vi "GUI_HTU_Laser_Control_Center.vi"() -> ()   [LabVIEW 2020]
uses:
  Shared/GUI_Template/GUI_master/tcp_new_data_event.ctl
  Shared/GUI_Template/GUI_master/tcp new data cluster.ctl
  GUI_TestStand/Fire button.ctl
panel:
  in  "Open Gaia South Shutter":bool caption="Open gaia North"
  in  "Open Gaia North Shutter":bool caption="Open gaia North"
  in  "Gaia shutter enable":bool caption="Enable gaia \nshutters"
  out "Laser on target":bool
  in  "GUIdevice 28":string="U_MI_FineFilters"
  in  "pos.Channel0::28":enum16{"1", "2", "3", "4", "5", "6"}(ring) caption="Fine Filters"
  in  "DO.Ch9::22":enum16{"off", "on"}(ring) caption="Aline2"
  in  "SoftwareVars.Ch1::22":enum16{"off", "on"}(ring) caption="Autopurge"
  in  "DO.Ch8::22":enum16{"off", "on"}(ring) caption="Aline 3"
  in  "DO.Ch7::22":enum16{"off", "on"}(ring) caption="DC Phos"
  in  "auto purge":bool=TRUE
  in  "purge":bool caption="Purge"
  in  "DO.Ch6::22":enum16{"off", "on"}(ring) caption="purge"
  out "AI_mean.Channel 1::27":dbl caption="Energy (nJ)" min=0.0 max=0.0 format="%.3f"
  out "AI_mean.Channel 0::27":dbl caption="Energy (nJ)" min=0.0 max=0.0 format="%.3f"
  in  "GUIdevice 27":string="U_VacuumGauge"
  out "ACavePressure":dbl format="%#_3g"
  out "BCavePressure":dbl format="%#_3g"
  in  "DigitalOutput.Channel 7::18":enum16{"off", "on"}(ring) caption="Visa9"
  in  "DigitalOutput.Channel 7::25":enum16{"off", "on"}(ring) caption="Visa1"
  in  "DigitalOutput.Channel 6::25":enum16{"off", "on"}(ring) caption="Visa2"
  in  "DigitalOutput.Channel 5::25":enum16{"off", "on"}(ring) caption="Visa3"
  in  "DigitalOutput.Channel 4::25":enum16{"off", "on"}(ring) caption="Visa4"
  in  "DigitalOutput.Channel 3::25":enum16{"off", "on"}(ring) caption="Visa5"
  in  "DigitalOutput.Channel 2::25":enum16{"off", "on"}(ring) caption="Visa6"
  in  "DigitalOutput.Channel 1::25":enum16{"off", "on"}(ring) caption="Visa7"
  in  "DigitalOutput.Channel 0::25":enum16{"off", "on"}(ring) caption="Visa8"
  in  "DigitalOutput.Channel 7::23":enum16{"off", "on"}(ring) caption="Aline1"
  in  "DO.Ch5::22":enum16{"off", "on"}(ring) caption="Beam \nDump"
  in  "DO.Ch4::22":enum16{"off", "on"}(ring) caption="Phos1"
  in  "DO.Ch3::22":enum16{"off", "on"}(ring) caption="MI Wedge"
  in  "DO.Ch2::22":enum16{"off", "on"}(ring) caption="Slit"
  in  "DO.Ch1::22":enum16{"off", "on"}(ring) caption="OAPin2"
  in  "GUIdevice 22":string="U_PLC"
  in  "Position.Channel 8::2":T1(ring) caption="TC phos"
  in  "pos.Channel1::5":enum16{"1", "2", "3", "4", "5", "6"}(ring) caption="HASO"
  in  "pos.Channel0::19":enum16{"1", "2", "3", "4", "5", "6"}(ring) caption="Grating \nCam"
  in  "GUIdevice 19":string="U_FilterWheel_02"
  in  "Delay.Ch B::10":dbl caption="OPening time" min=0.0 max=0.1 format="%#_6p"
  in  "Amplitude.Ch AB::10":dbl caption="Amplitude Jet trigger" min=0.5 max=5.0 format="%.1f"
  in  "DO.Ch10::22":enum16{"off", "on"}(ring) caption="CTR"
  in  "GUIdevice 17":string="U_Hexapod"
  in  "Position.Channel 9::1":T1(ring) caption="Amp 4 dump"
  in  "Position.Channel 10::1":T1(ring) caption="Revo-South Shutter"
  in  "Position.Channel 7::1":T1(ring) caption="Gaia Beamblock 2-North"
  in  "Position.Channel 8::1":T1(ring) caption="Gaia Beamblock 2-South"
  out "Delay.Ch B::10":dbl caption="Opening \ntime (s)" min=0.0 max=0.1 format="%#_6p"
  in  "Set opening time (s)":dbl
  in  "Jet enable":bool caption="Jet Enable"
  in  "pos.Channel3::5":enum16{"1", "2", "3", "4", "5", "6"}(ring) caption="Probe"
  in  "pos.Channel2::5":enum16{"1", "2", "3", "4", "5", "6"}(ring) caption="Ghost\npulsed"
  in  "AnalogOutput.Channel 1::8":dbl caption="Pressure Control Voltage (V)" min=0.0 max=10.0
  in  "Position.Axis 3::7":dbl caption="Jet_Z" min=0.0 max=25.0
  in  "Position.Axis 2::7":dbl caption="Jet_Y" min=-25.0 max=0.0
  in  "Position.Axis 1::7":dbl caption="Jet_X" min=0.0 max=25.0
  in  "pos.Channel0::5":enum16{"1", "2", "3", "4", "5", "6"}(ring) caption="Coarse Filters"
  in  "Position.Channel 6::1":T1(ring) caption="Gaia Beamblock 3-North"
  in  "Position.Channel 5::1":T1(ring) caption="Gaia Beamblock 4-North"
  in  "Position.Channel 4::1":T1(ring) caption="Gaia Stop South"
  in  "Position.Channel 3::1":T1(ring) caption="Gaia Stop North"
  in  "Position.Channel 2::1":T1(ring) caption="Gaia Beamblock 3-South"
  in  "Position.Channel 1::1":T1(ring) caption="Gaia Beamblock 4-South"
  in  "GUIdevice 8":string="U_HP_Daq"
  in  "GUIdevice 5":string="U_FilterWheel_01"
  in  "Fire Button":T2=TRUE
  out "error IO 2":errorcluster
  out "Amplitude.Ch AB::10":dbl caption="Amplitude\n Jet trigger" min=0.5 max=5.0 format="%.1f"
  out "fire::10":string
  out "tcp data event":T3
  in  "UDP error message":string
  in  "GUIdevice 7":string="U_ESP_JetXYZ"
  in  "GUIdevice 2":string="U_1Wire_Bcave"
  in  "GUIdevice 10":string="U_DG645_ShotControl"
  in  "GUIdevice 1":string="U_1Wire_148"
  in  "Step size":dbl min=-22.0 max=22.0 format="%.5f"
  in  "wangle::17":dbl caption="w" min=-7.5 max=7.5 step=0.01 format="%.5f"
  in  "vangle::17":dbl caption="v" min=-7.5 max=7.5 step=0.01 format="%.5f"
  in  "uangle::17":dbl caption="u" min=-7.5 max=7.5 step=0.01 format="%.5f"
  in  "ypos::17":dbl caption="y" min=-24.0 max=24.0 step=0.01 format="%.5f"
  in  "zpos::17":dbl caption="z" min=-10.0 max=10.0 step=0.01 format="%.5f"
  in  "xpos::17":dbl caption="x" min=-20.0 max=20.0 step=0.01 format="%.5f"
  in  "Jet trigger":bool caption="Jet Trigger"
  in  "Delay.Ch C::10":dbl caption="Jet timing (s)" min=-0.1 max=0.1 format="%#_6p"
  in  "stop":bool
  # "HTU CONTROL CENTER"
  # "GAIA Flippers"
  # "B-Cave Laser Status"
  # "Jet Stages"
  # "Energy"
  # "Mode Imager"
  # "Jet timing"
  # "Hexapod"
  # "\"+x\" is laser propagation direction\n\"+y\" is toward parking lot\n\"+z\" is up"
  # "Extra Flippers"
  # "Valve Control"
  # "Filters"
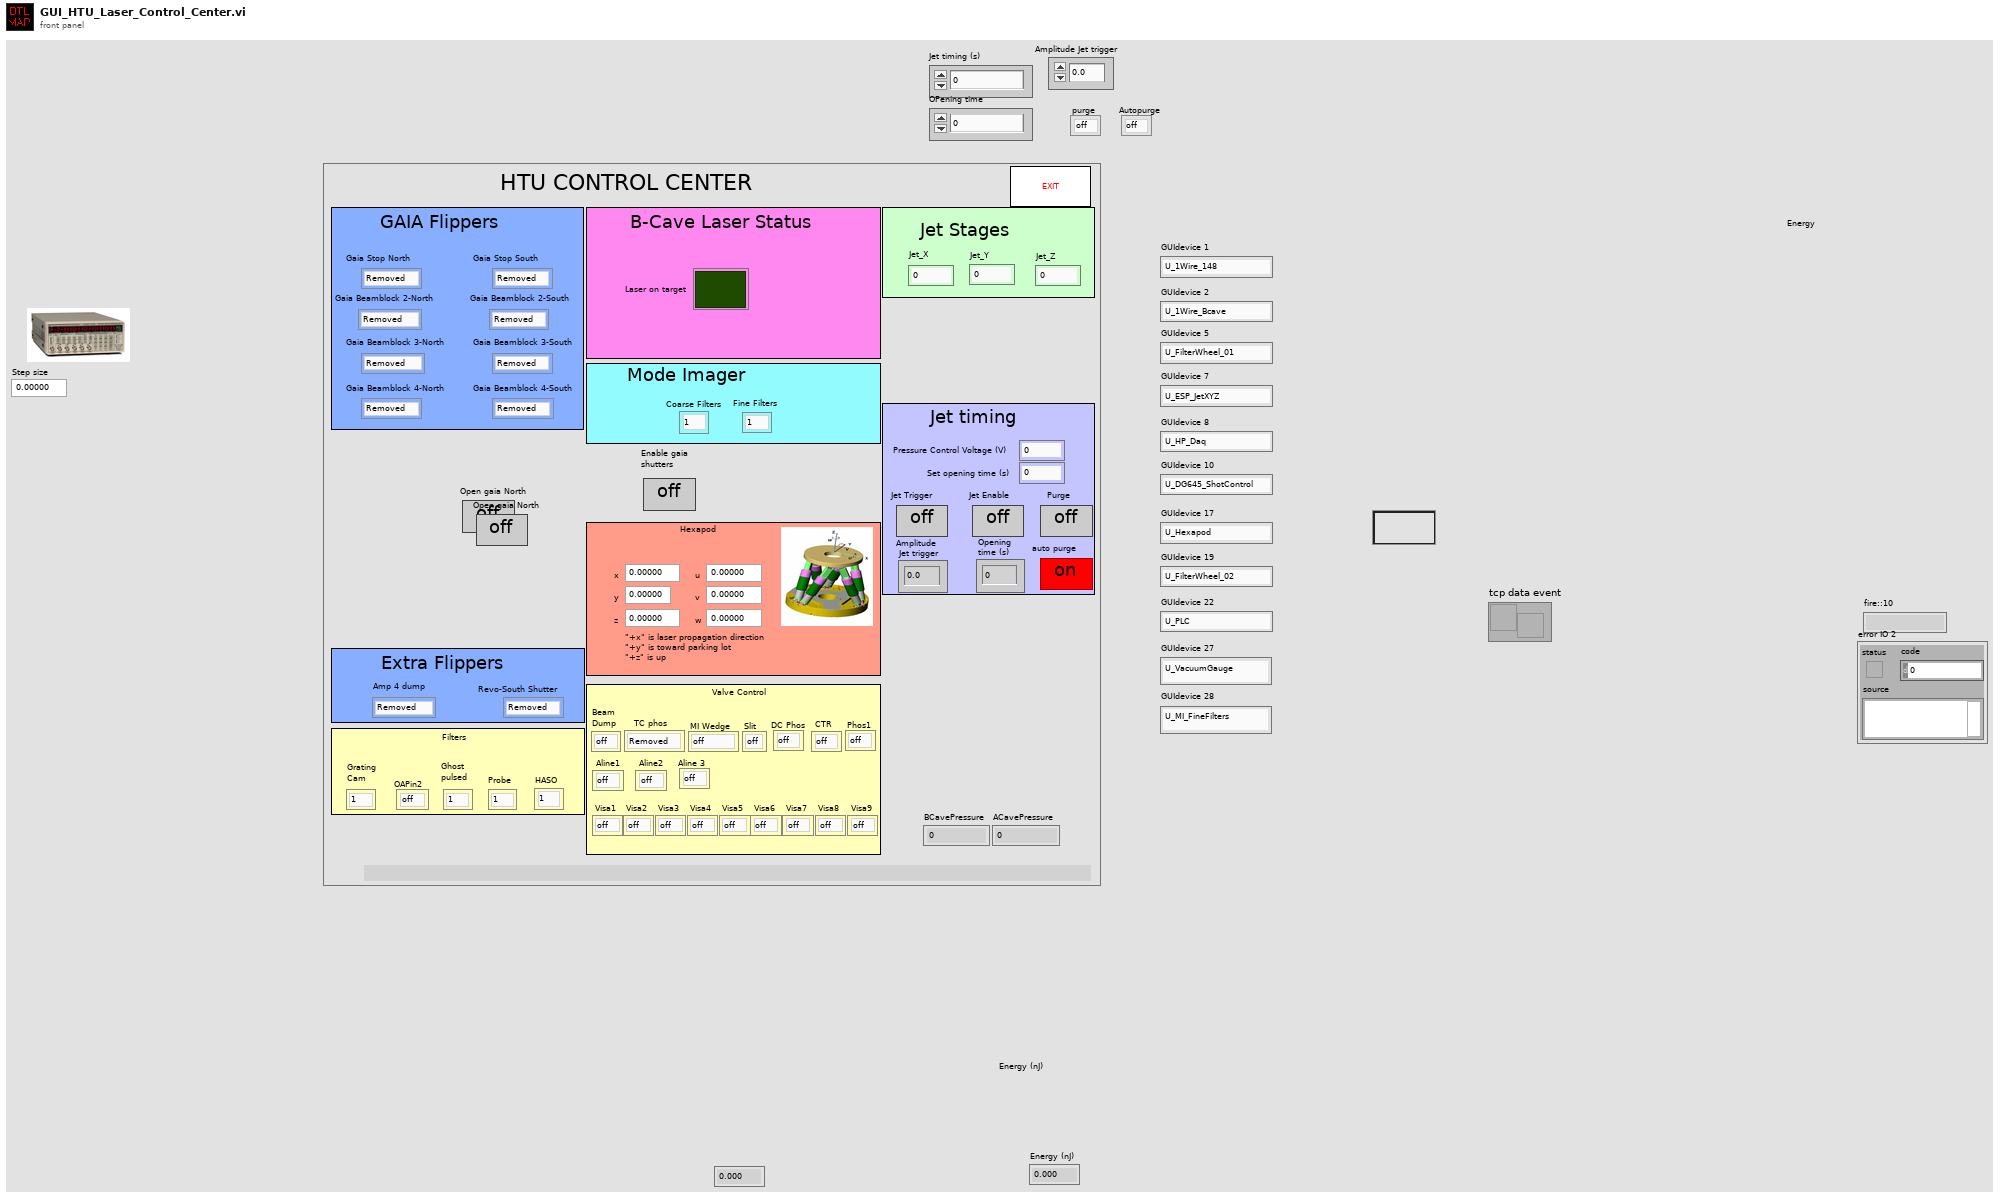
[diagram p1: front panel]
types:
  T1 = enum16{"Removed", "Inserted", "Unknown", "Moving"}
  T2 = typedef "Fire button.ctl" = bool
  T3 = typedef "tcp_new_data_event.ctl" = refnum<user-event>
  T4 = typedef "tcp new data cluster.ctl" = cluster{"EventEnum":enum16{"new data", "connection status update"}, "Device name":string}
  T5 = enum32{"invalid app kind", "Development System", "Run Time System", "Student Edition", "Embedded LabVIEW", "Evaluation", "Custom"}
  T6 = enum32{"Invalid", "Standard", "Closed", "Hidden", "Minimized", "Maximized"}
  T7 = cluster{"Core":cluster{"Current VI Reference":refnum<vi>, "Close Panel on Exit?":bool}, "BCavePressure":dbl, "ACavePressure":dbl, "Jet trigger":bool, "Jet probe stage tck":u32, "Tik2":u32, "Fire Continues Allowed":bool, "Jet enable":bool, "Wedge enable":bool, "Phosphor enable":bool, "jet status tck":i32, "purge":bool, "auto purge":bool, "IR beam on target":bool, "Gaia shutter enable":bool, "Open Gaia north shutter":bool, "Open Gaia north shutter":bool}
  T8 = cluster{"Current VI Reference":refnum<vi>, "Close Panel on Exit?":bool}
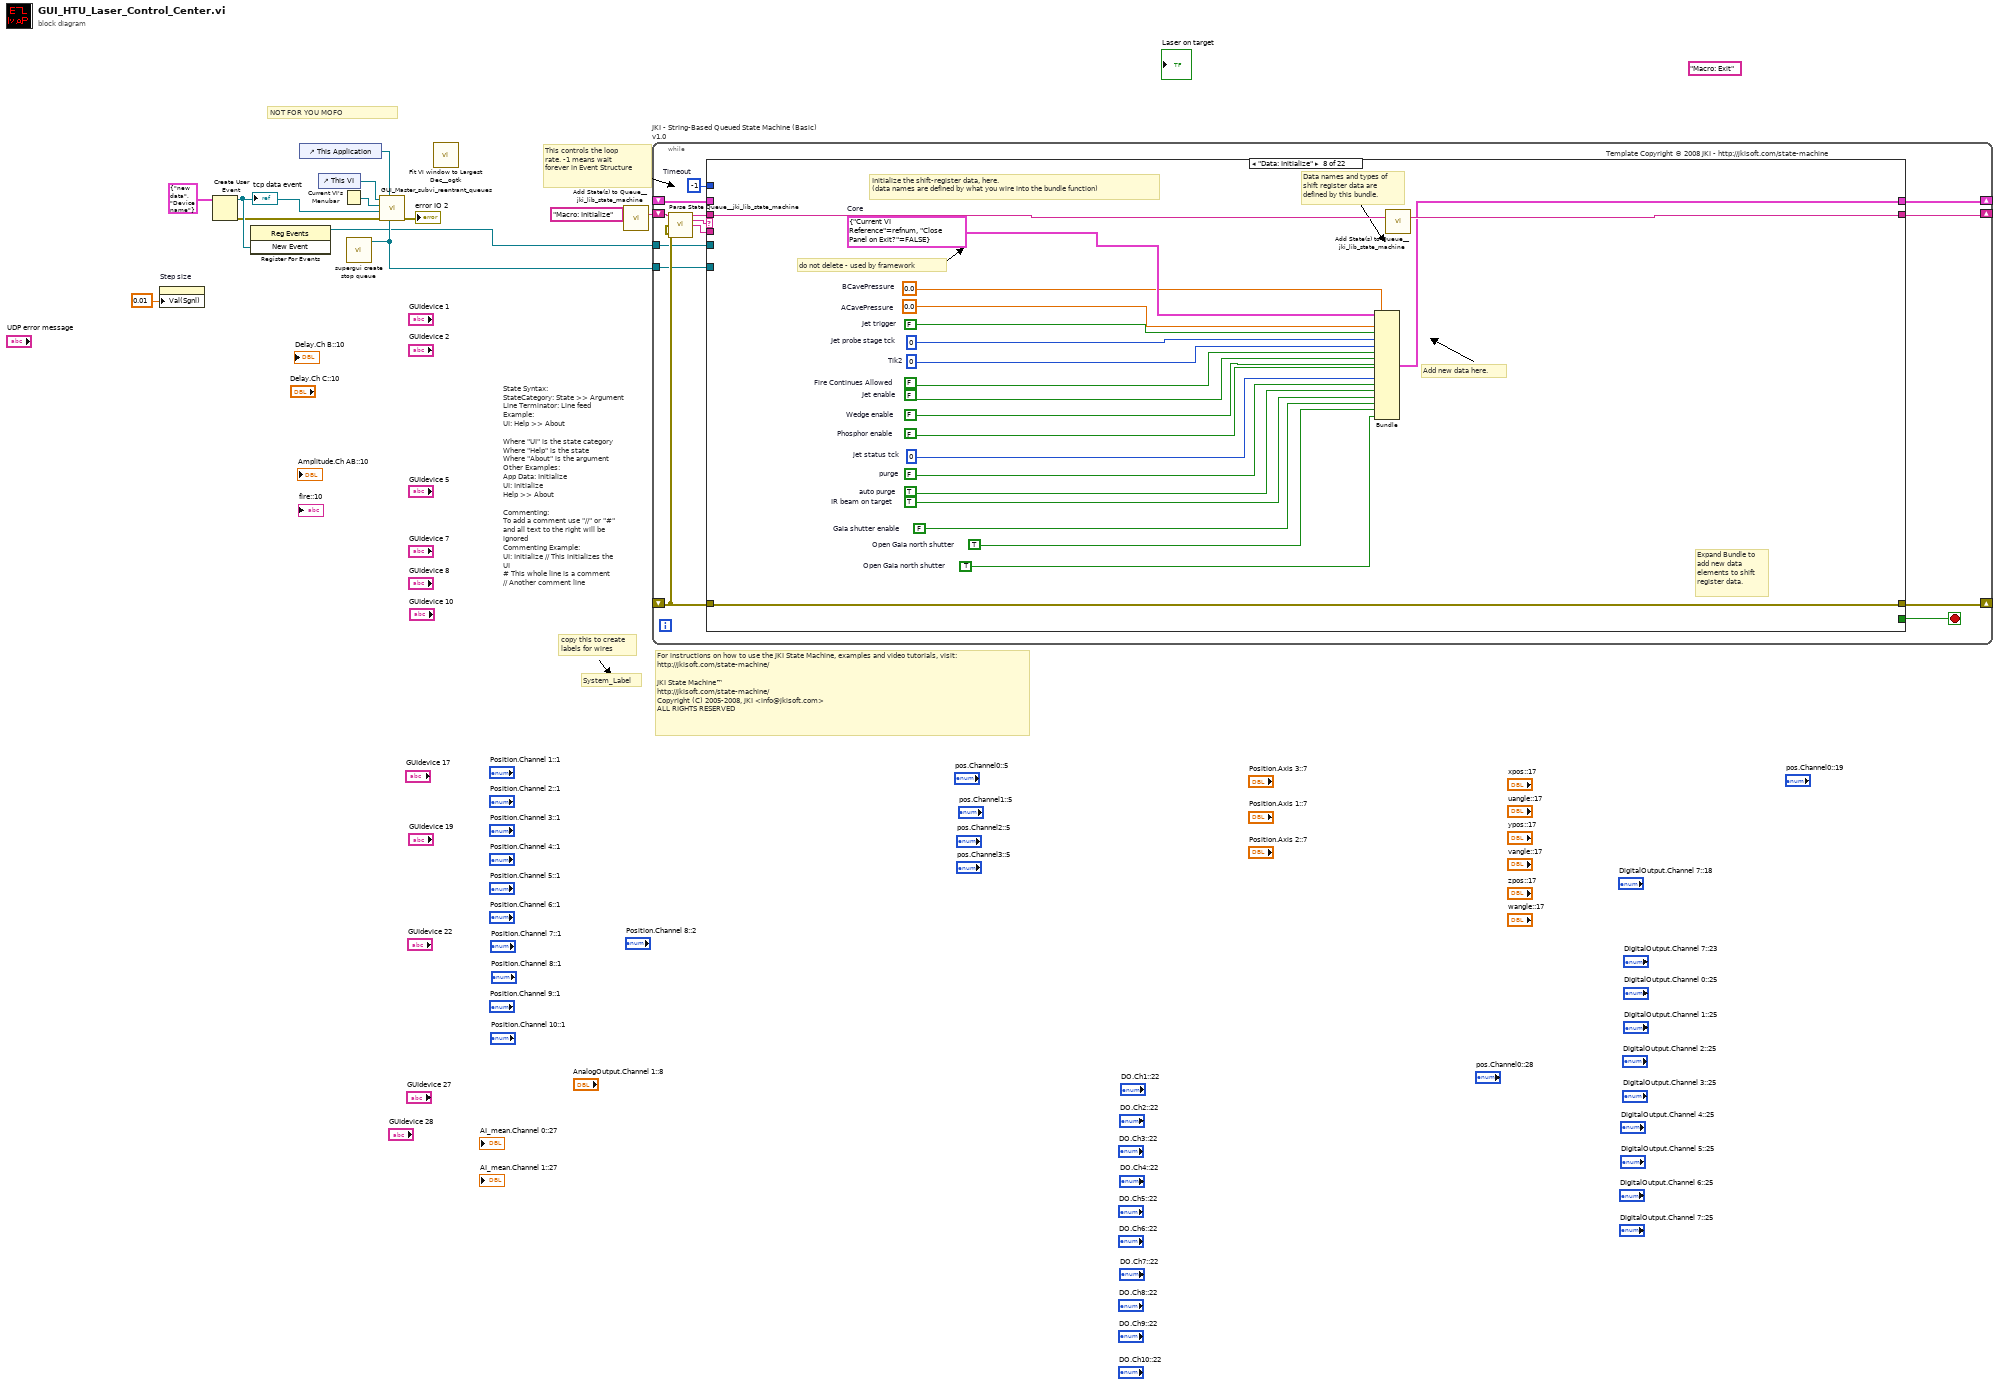
[diagram p0: block diagram]
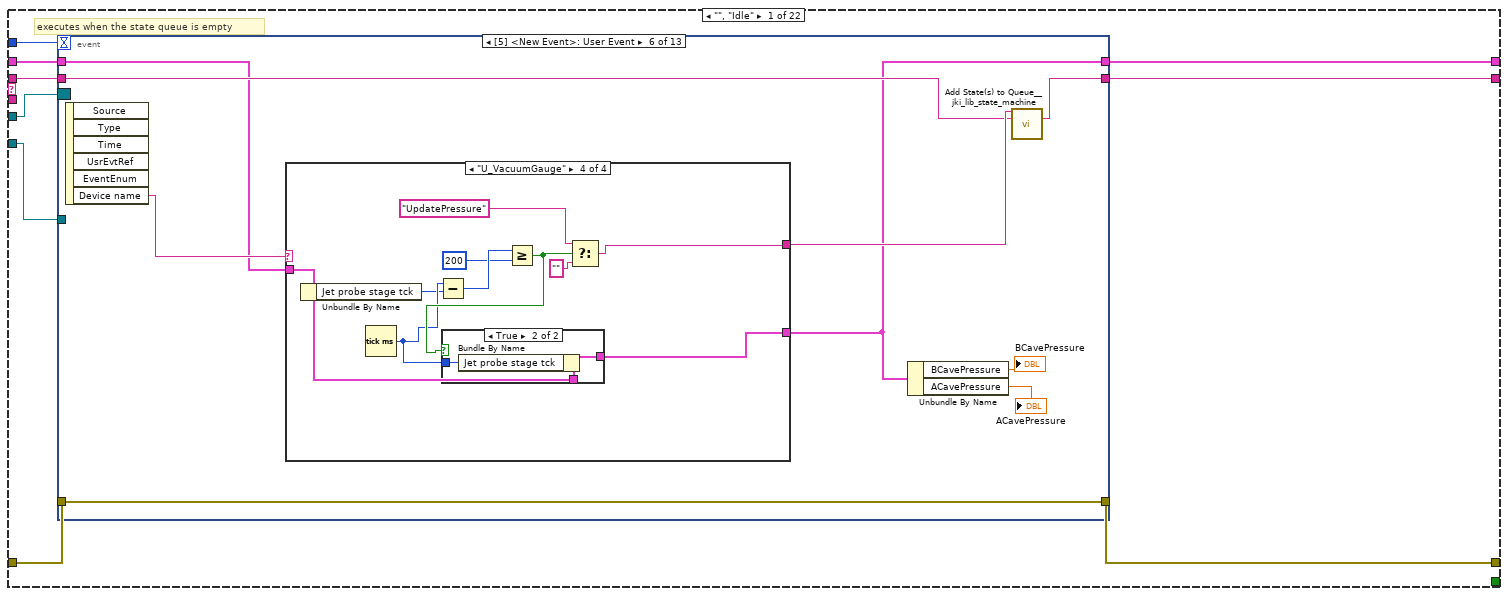
[diagram p2: hidden frame]
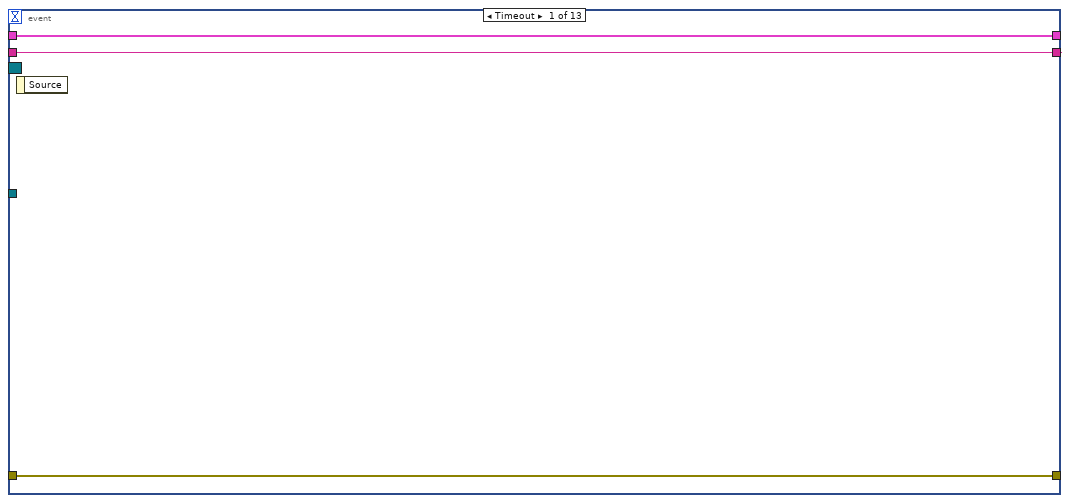
[diagram p3: hidden frame]
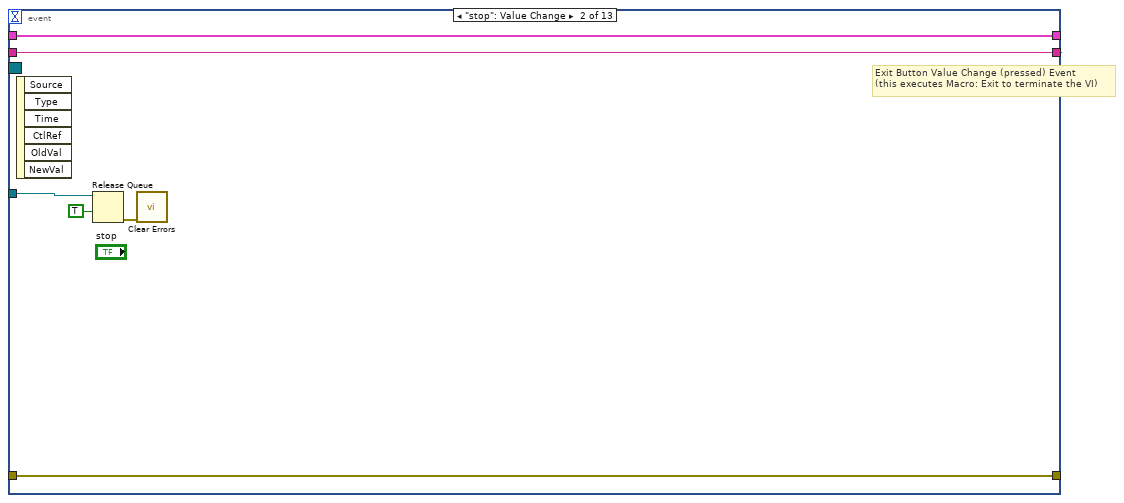
[diagram p4: hidden frame]
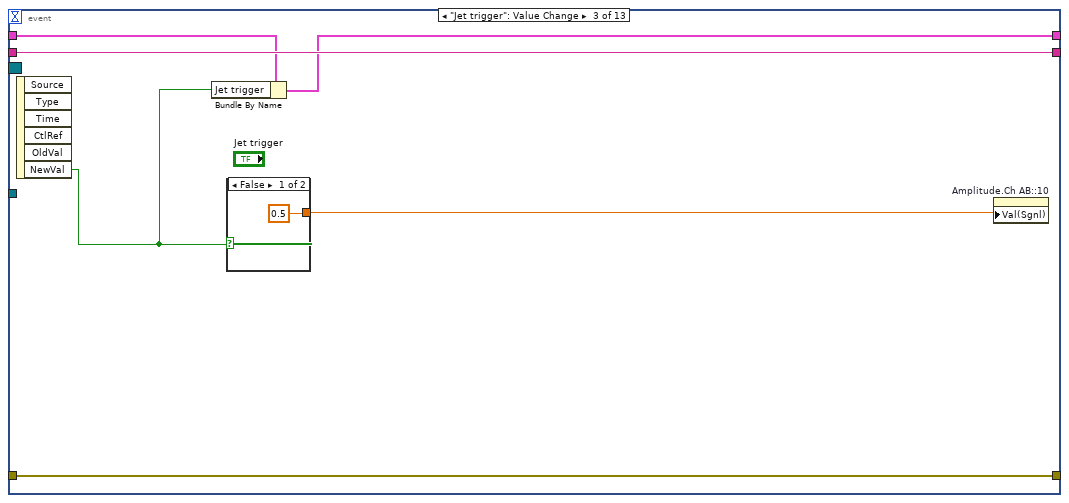
[diagram p5: hidden frame]
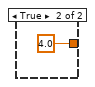
[diagram p6: hidden frame]
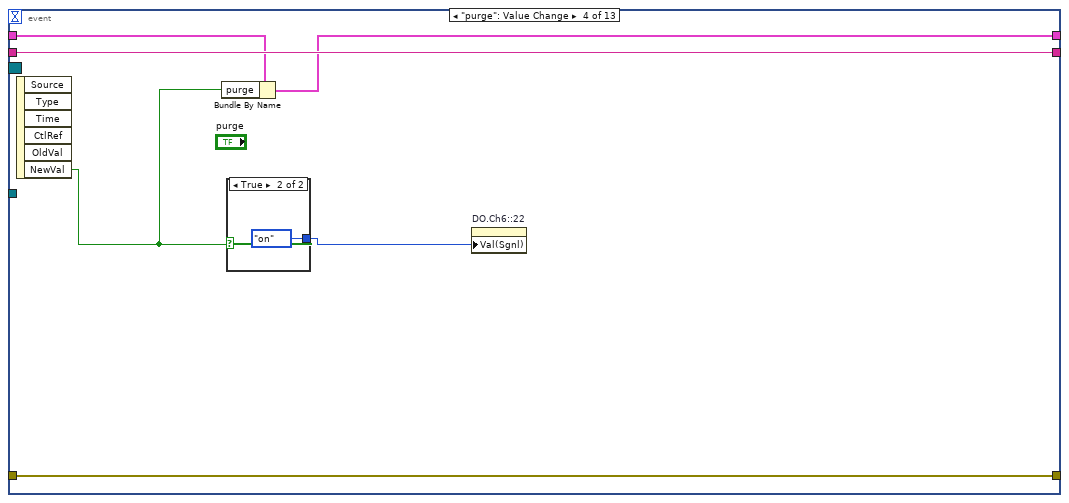
[diagram p7: hidden frame]
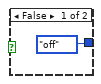
[diagram p8: hidden frame]
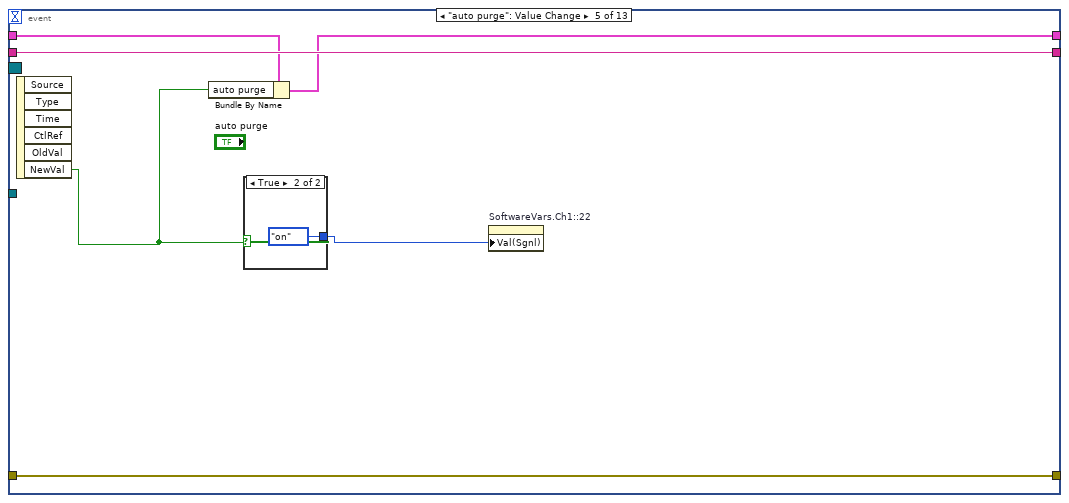
[diagram p9: hidden frame]
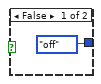
[diagram p10: hidden frame]
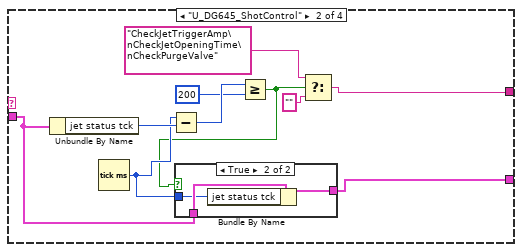
[diagram p12: hidden frame]
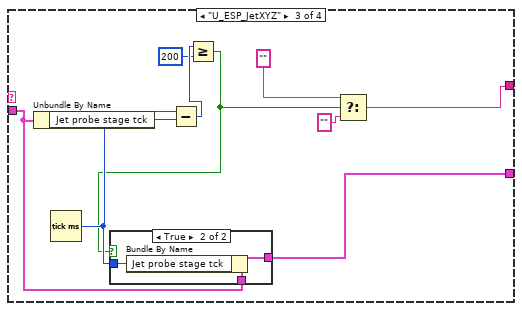
[diagram p14: hidden frame]
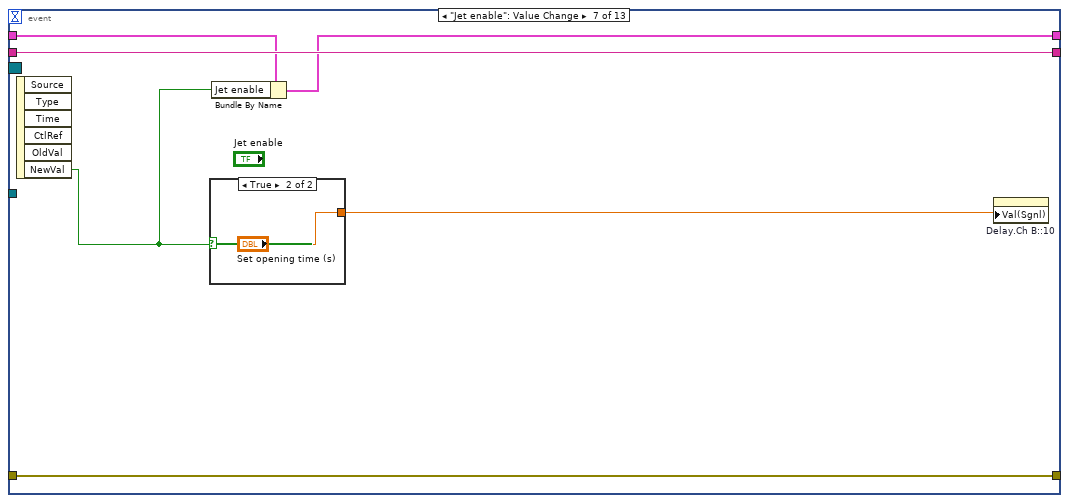
[diagram p17: hidden frame]
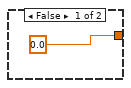
[diagram p18: hidden frame]
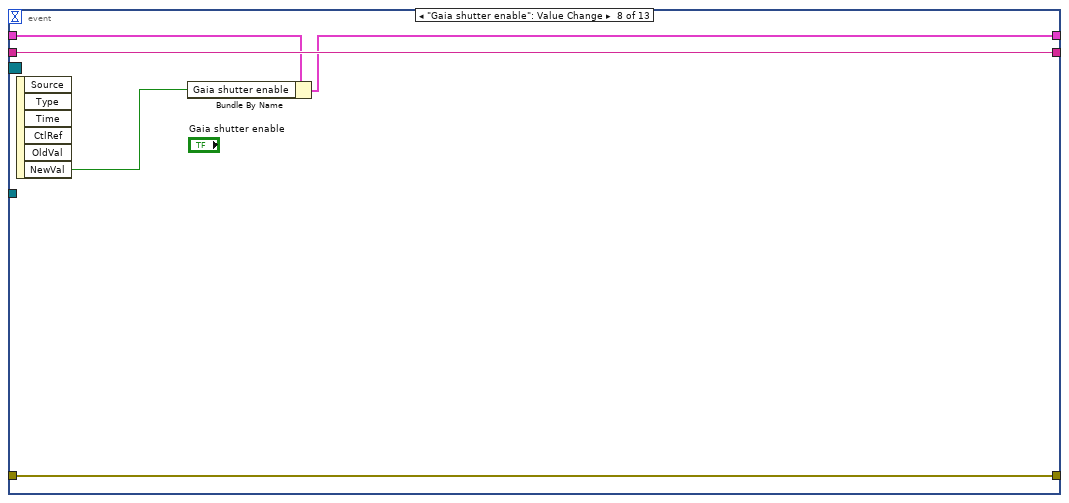
[diagram p19: hidden frame]
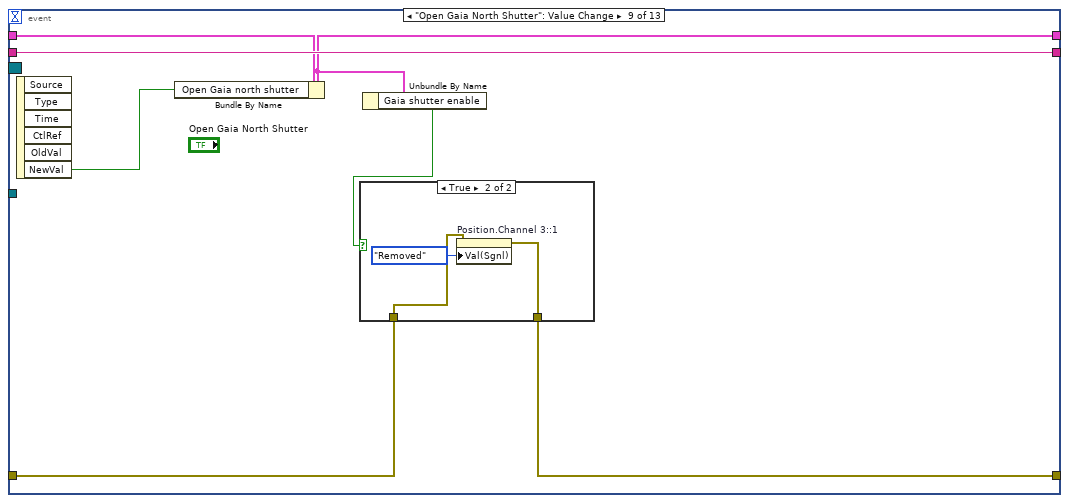
[diagram p20: hidden frame]
diagram:
  (unwired) "Macro: Exit"
  # "For instructions on how to use the JKI State Machine, examples and video tutorials, visit:\nhttp://jkisoft.com/state-machine/\n\nJKI State Machine™\nhttp://jkisoft.com/state-machine/\nCopyright (C) 2005-2008, JKI <info@jkisoft.com>\nALL RIGHTS RESERVED"
  # "State Syntax:\nStateCategory: State >> Argument\nLine Terminator: Line feed\nExample:\nUI: Help >> About\n\nWhere \"UI\" is the state category\nWhere \"Help\" is the state\nWhere \"About\" is the argument\nOther Examples:\nApp Data: Initialize\nUI: Initialize\nHelp >> About\n\nCommenting:\nTo add a comment use \"//\" or \"#\" and all text to the right will be ignored\nCommenting Example:\nUI: Initialize // This initializes the UI\n# This whole line is a comment\n// Another comment line"
  # "copy this to create labels for wires"
  # "This controls the loop rate. -1 means wait forever in Event Structure"
  # "System_Label"
  # "NOT FOR YOU MOFO"
  n1 = property on="Step size" class="DigNum (strict)"("Val(Sgnl)"=0.01 ("Value (Signaling)")) -> ()  [unwired: 2 in, 2 out]
  n2 = Create User Event(user event datatype=T4 {"EventEnum"=enum."new data", "Device name"="Device name"} ("New Event")) -> (user event=w11:refnum<user-event>, error out=w10:errorcluster)  [unwired: 1 in]
  "tcp data event" <- w11
  n3 = register-events(w11) -> (reference out=w1:refnum<event-registration>)  [unwired: 2 in, 1 out]
  n4 = control-ref of="This Application"() -> (w12:refnum<vi>)
  n5 = control-ref of="This VI"() -> (w5:refnum<vi>)
  n6 = Current VI's Menubar() -> (w8:refnum<k9>)
  n7 = call "supergui create stop queue.vi"() -> ("STOP Queue out"=w2:refnum<queue>)  [unwired: 11 in]
  n8 = call "GUI_Master_subvi_reentrant_queues.vi"("STOP Queue in"=w2, "This Application"=w12, "error in (no error)"=w10, "tcp data event"=w11, "Caller menu reference"=w8, "Caller VI ref"=w5) -> ("error out"=→"error IO 2":errorcluster)  [unwired: 5 in]
  n9 = call <userlib>:"Fit VI window to Largest Dec__ogtk.vi"() -> ()  [unwired: 6 in, 2 out]
  n10 = call <vilib>:"Add State(s) to Queue__jki_lib_state_machine.vi"("State(s) in (\"\")"="Macro: Initialize") -> ("States Out"=w3:string)  [unwired: 14 in]
  n11 = while "JKI - String-Based Queued State Machine (Basic) v1.0" {
    shift-right: [w18] -> _
    shift-left: _ -> [w17]
    shift-right: [w21] -> _
    shift-left: _ -> [w15]
    shift-right: [w20] -> _
    shift-left: w3 -> [w22]
    tunnel: w1 -> [w14]
    tunnel: w2 -> [w13]
    stop <- w19 stop-if-true
    w16 = -1  # Timeout
    # "Template Copyright © 2008 JKI - http://jkisoft.com/state-machine"
    n12 = call <vilib>:"Parse State Queue__jki_lib_state_machine.vi"("State Queue"=w22, "Error In (no error)"=w15) -> ("Remaining States"=w24:string, "Current State"=w25:string, "Arguments"=w23:string)  [unwired: 11 in]
    n13 = case shown="\"Data: Initialize\"" w25 {
      selector: w25 -> [_ _ w181 _ _ _ _ _ _ _ _ _ _ _ _ _ _ _ _ _ _ _]
      tunnel: w24 -> [w34 w180 w185 w203 w209 w214 w218 w239 w245 w249 w253 w259 w270 w296 w301 w311 w315 w321 w334 w350 w365 w417]
      tunnel: w23 -> [_ _ _ _ _ _ _ _ _ _ _ w254 w264 _ _ _ _ _ _ _ _ _]
      tunnel: w17 -> [w32 w177 w183 w194 w206 w212 w215 _ w240 w246 w251 w257 w266 w293 w298 w308 w312 w319 w331 w347 w361 w406]
      tunnel: [w31 w178 w187 w200 errorcluster {"status"=FALSE, "code"=0, "source"=""} ("error out") w211 w216 w236 w241 w247 w250 w255 w267 w294 w299 w309 w313 w316 w332 w348 w358 w407] -> w21
      tunnel: w15 -> [w30 w178 w186 w200 w205 w211 w216 w236 w242 w247 w250 w256 w268 w294 w299 w309 w313 w317 w332 w348 w359 w407]
      tunnel: [w33 w179 w184 w202 w208 w213 w217 w238 w244 w248 w252 w258 w269 w295 w300 w310 w314 w320 w333 w349 w364 w416] -> w20
      tunnel: [_ _ _ _ _ TRUE _ _ _ _ _ _ _ _ _ _ _ _ _ _ _ _] -> w19
      tunnel: [w26 w177 w183 w201 w206 w212 w215 w237 w240 w246 w251 w257 w266 w293 w298 w308 w312 w319 w330 w346 w360 w405] -> w18
      tunnel: w16 -> [w29 _ _ _ _ _ _ _ _ _ _ _ _ _ _ _ _ _ _ _ _ _]
      tunnel: w14 -> [w28 _ _ _ _ _ _ _ _ _ _ _ _ _ _ _ _ _ _ _ _ _]
      tunnel: w13 -> [w27 _ _ _ _ _ _ _ _ _ _ _ _ _ _ _ _ _ _ _ _ _]
      frame "", "Idle" {
        # "executes when the state queue is empty"
        n14 = event shown="[5] <New Event>: User Event" {
          selector: w28 -> [_ _ _ _ _ _ _ _ _ _ _ _ _]
          dyn-events: _ -> [_ _ _ _ _ _ _ _ _ _ _ _ _]
          timeout: w29 -> [_ _ _ _ _ _ _ _ _ _ _ _ _]
          tunnel: w34 -> [w38 w46 w52 w60 w68 w76 w128 w135 w142 w155 w163 w168 w176]
          tunnel: [w37 w45 w52 w60 w68 w75 w128 w135 w142 w155 w164 w168 w175] -> w33
          tunnel: w32 -> [w35 w43 w51 w59 w67 w74 w127 w134 w141 w154 w166 w169 w173]
          tunnel: [w36 w44 w47 w56 w65 w79 w123 w131 w136 w149 w165 w167 w174] -> w31
          tunnel: w30 -> [w36 w44 w47 w56 w65 w79 w123 w131 w137 w150 w165 w167 w174]
          tunnel: [w35 w43 w50 w58 w66 w73 w126 w133 w139 w152 w166 w169 w173] -> w26
          tunnel: w27 -> [_ w40 _ _ _ _ _ _ _ _ _ _ _]
          event Timeout {
            n15 = event-data() -> ()  [unwired: 1 in, 1 out]
            n16 = call <vilib>:"Add State(s) to Queue__jki_lib_state_machine.vi"("State(s) in (\"\")"=w38) -> ("States Out"=w37:string)  [unwired: 14 in]
          }
          event "stop": Value Change {
            # "Exit Button Value Change (pressed) Event\n(this executes Macro: Exit to terminate the VI)"
            n17 = event-data() -> ()  [unwired: 1 in, 6 out]
            n18 = Release Queue(queue=w40, force destroy? (F)=TRUE) -> (error out=w41:errorcluster)  [unwired: 1 in, 2 out]
            n19 = call <vilib>:"Clear Errors.vi"("error in (no error)"=w41) -> ()  [unwired: 5 in, 2 out]
            n20 = call <vilib>:"Add State(s) to Queue__jki_lib_state_machine.vi"("State(s) in Front (\"\")"="Macro: Exit", "State(s) in (\"\")"=w46) -> ("States Out"=w45:string)  [unwired: 13 in]
          }
          event "Jet trigger": Value Change {
            n21 = event-data() -> ("NewVal"=w49:bool)  [unwired: 1 in, 5 out]
            n22 = Bundle By Name(cluster=w51, "Jet trigger"=w49) -> (w50:T7)
            n23 = case shown="False" w49 {
              tunnel: [0.5 ("Amplitude.Ch CD::10") 4.0 ("Amplitude.Ch CD::10")] -> w48
              frame False {
              }
              frame True {
              }
            }
            n24 = property on="Amplitude.Ch AB::10" class="DigNum (strict)"("Val(Sgnl)"=w48) -> ()  [unwired: 2 in, 2 out]
          }
          event "purge": Value Change {
            n25 = event-data() -> ("NewVal"=w57:bool)  [unwired: 1 in, 5 out]
            n26 = Bundle By Name(cluster=w59, "purge"=w57) -> (w58:T7)
            n27 = case shown="True" w57 {
              tunnel: [enum16{"off", "on"}."off" ("Value (Signaling)") enum16{"off", "on"}."on" ("Value (Signaling)")] -> w55
              frame False {
              }
              frame True {
              }
            }
            n28 = property on="DO.Ch6::22" class="Enum (strict)"("Val(Sgnl)"=w55) -> ()  [unwired: 2 in, 2 out]
          }
          event "auto purge": Value Change {
            n29 = event-data() -> ("NewVal"=w63:bool)  [unwired: 1 in, 5 out]
            n30 = Bundle By Name(cluster=w67, "auto purge"=w63) -> (w66:T7)
            n31 = case shown="True" w63 {
              tunnel: [enum16{"off", "on"}."off" ("Value (Signaling)") enum16{"off", "on"}."on" ("Value (Signaling)")] -> w64
              frame False {
              }
              frame True {
              }
            }
            n32 = property on="SoftwareVars.Ch1::22" class="Enum (strict)"("Val(Sgnl)"=w64) -> ()  [unwired: 2 in, 2 out]
          }
          event User Event {
            n33 = event-data() -> ("Device name"=w78:string)  [unwired: 1 in, 5 out]
            n34 = case shown="\"U_VacuumGauge\"" w78 {
              tunnel: [_ w84 w96 w109] -> w77
              tunnel: w74 -> [w80 w82 w100 w111]
              tunnel: [w80 w81 w99 w110] -> w73
              frame "False", Default {
              }
              frame "U_DG645_ShotControl" {
                n35 = Unbundle By Name(w82) -> ("jet status tck"=w90:i32)
                n36 = Tick Count (ms)() -> (millisecond timer value=w86:u32)
                n37 = Subtract(x=w86, y=w90) -> (x-y=w89:u32)
                n38 = Greater Or Equal?(x=w89, y=u32 200 ("x")) -> (x >= y?=w85:bool)
                n39 = case shown="True" w85 {
                  tunnel: [w91 w94] -> w81
                  tunnel: w82 -> [w91 w93]
                  tunnel: w86 -> [_ w92]
                  frame False {
                  }
                  frame True {
                    n40 = Bundle By Name(cluster=w93, "jet status tck"=w92) -> (w94:T7)
                  }
                }
                n41 = Select(t="CheckJetTriggerAmp\nCheckJetOpeningTime\nCheckPurgeValve", s=w85, f="") -> (s? t:f=w84:string)
              }
              frame "U_ESP_JetXYZ" {
                n42 = Unbundle By Name(w100) -> ("Jet probe stage tck"=w104:u32)
                n43 = Tick Count (ms)() -> (millisecond timer value=w101:u32)
                n44 = Subtract(x=w101, y=w104) -> (x-y=w103:u32)
                n45 = Greater Or Equal?(x=w103, y=u32 200 ("x")) -> (x >= y?=w95:bool)
                n46 = case shown="True" w95 {
                  tunnel: [w105 w108] -> w99
                  tunnel: w100 -> [w105 w107]
                  tunnel: w101 -> [_ w106]
                  frame False {
                  }
                  frame True {
                    n47 = Bundle By Name(cluster=w107, "Jet probe stage tck"=w106) -> (w108:T7)
                  }
                }
                n48 = Select(t="", s=w95, f="") -> (s? t:f=w96:string)
              }
              frame "U_VacuumGauge" {
                n49 = Unbundle By Name(w111) -> ("Jet probe stage tck"=w115:u32)
                n50 = Tick Count (ms)() -> (millisecond timer value=w117:u32)
                n51 = Subtract(x=w117, y=w115) -> (x-y=w116:u32)
                n52 = Greater Or Equal?(x=w116, y=u32 200 ("x")) -> (x >= y?=w118:bool)
                n53 = case shown="True" w118 {
                  tunnel: [w119 w122] -> w110
                  tunnel: w111 -> [w119 w121]
                  tunnel: w117 -> [_ w120]
                  frame False {
                  }
                  frame True {
                    n54 = Bundle By Name(cluster=w121, "Jet probe stage tck"=w120) -> (w122:T7)
                  }
                }
                n55 = Select(t="UpdatePressure", s=w118, f="") -> (s? t:f=w109:string)
              }
            }
            n56 = Unbundle By Name(w73) -> ("BCavePressure"=→"BCavePressure":dbl, "ACavePressure"=→"ACavePressure":dbl)
            n57 = call <vilib>:"Add State(s) to Queue__jki_lib_state_machine.vi"("State(s) in Front (\"\")"=w77, "State(s) in (\"\")"=w76) -> ("States Out"=w75:string)  [unwired: 13 in]
          }
          event "Jet enable": Value Change {
            n58 = event-data() -> ("NewVal"=w125:bool)  [unwired: 1 in, 5 out]
            n59 = case shown="True" w125 {
              tunnel: [0.0 ("opening Time") "Set opening time (s)"] -> w124
              frame False {
              }
              frame True {
              }
            }
            n60 = Bundle By Name(cluster=w127, "Jet enable"=w125) -> (w126:T7)
            n61 = property on="Delay.Ch B::10" class="DigNum (strict)"("Val(Sgnl)"=w124) -> ()  [unwired: 2 in, 2 out]
          }
          event "Gaia shutter enable": Value Change {
            n62 = event-data() -> ("NewVal"=w132:bool)  [unwired: 1 in, 5 out]
            n63 = Bundle By Name(cluster=w134, "Gaia shutter enable"=w132) -> (w133:T7)
          }
          event "Open Gaia North Shutter": Value Change {
            n64 = event-data() -> ("NewVal"=w140:bool)  [unwired: 1 in, 5 out]
            n65 = Bundle By Name(cluster=w141, "Open Gaia north shutter"=w140) -> (w139:T7)
            n66 = Unbundle By Name(w139) -> ("Gaia shutter enable"=w138:bool)
            n67 = case shown="True" w138 {
              tunnel: w137 -> [w144 w147]
              tunnel: [w143 w146] -> w136
              frame False {
                n68 = property on="Position.Channel 3::1" class="Enum (strict)"(error in=w144, "Val(Sgnl)"=T1."Inserted" ("Value (Signaling)")) -> (error out=w143:errorcluster)  [unwired: 1 in, 1 out]
              }
              frame True {
                n69 = property on="Position.Channel 3::1" class="Enum (strict)"(error in=w147, "Val(Sgnl)"=T1."Removed" ("Value (Signaling)")) -> (error out=w146:errorcluster)  [unwired: 1 in, 1 out]
              }
            }
          }
          event "Open Gaia South Shutter": Value Change {
            n70 = event-data() -> ("NewVal"=w153:bool)  [unwired: 1 in, 5 out]
            n71 = Bundle By Name(cluster=w154, "Open Gaia north shutter"=w153) -> (w152:T7)
            n72 = Unbundle By Name(w152) -> ("Gaia shutter enable"=w151:bool)
            n73 = case shown="True" w151 {
              tunnel: w150 -> [w157 w160]
              tunnel: [w156 w159] -> w149
              frame False {
                n74 = property on="Position.Channel 3::1" class="Enum (strict)"(error in=w157, "Val(Sgnl)"=T1."Inserted" ("Value (Signaling)")) -> (error out=w156:errorcluster)  [unwired: 1 in, 1 out]
              }
              frame True {
                n75 = property on="Position.Channel 3::1" class="Enum (strict)"(error in=w160, "Val(Sgnl)"=T1."Removed" ("Value (Signaling)")) -> (error out=w159:errorcluster)  [unwired: 1 in, 1 out]
              }
            }
          }
          event Value Change {
            n76 = event-data() -> ()  [unwired: 1 in, 6 out]
            n77 = call <vilib>:"Add State(s) to Queue__jki_lib_state_machine.vi"("State(s) in Front (\"\")"="Action: Fire" ("State(s) in Front (\"\")"), "State(s) in (\"\")"=w163) -> ("States Out"=w164:string)  [unwired: 13 in]
          }
          event "Step size": Value Change {
            n78 = event-data() -> ("NewVal"=w170:dbl)  [unwired: 1 in, 5 out]
            n79 = property on="uangle::17" class="DigNum (strict)"("Increment"=w170) -> ()  [unwired: 2 in, 2 out]
            n80 = property on="vangle::17" class="DigNum (strict)"("Increment"=w170) -> ()  [unwired: 2 in, 2 out]
            n81 = property on="xpos::17" class="DigNum (strict)"("Increment"=w170) -> ()  [unwired: 2 in, 2 out]
            n82 = property on="zpos::17" class="DigNum (strict)"("Increment"=w170) -> ()  [unwired: 2 in, 2 out]
            n83 = property on="wangle::17" class="DigNum (strict)"("Increment"=w170) -> ()  [unwired: 2 in, 2 out]
            n84 = property on="ypos::17" class="DigNum (strict)"("Increment"=w170) -> ()  [unwired: 2 in, 2 out]
          }
          event Panel Close? {
            # "Discard the event because we'll close the front panel ourselves in Macro: Exit"
            # "Close Panel button (pressed) Event\n(this executes Macro: Exit to terminate the VI)"
            n85 = event-data() -> ()  [unwired: 1 in, 1 out]
            n86 = event-data("Discard?"=TRUE) -> ()  [unwired: 1 in, 1 out]
            n87 = call <vilib>:"Add State(s) to Queue__jki_lib_state_machine.vi"("State(s) in Front (\"\")"="Macro: Exit", "State(s) in (\"\")"=w176) -> ("States Out"=w175:string)  [unwired: 13 in]
          }
        }
      }
      frame "---------- Core ----------" {
        # "Do not put any code in this frame.\n(it is a separator no-op)"
        n88 = call <vilib>:"Add State(s) to Queue__jki_lib_state_machine.vi"("State(s) in (\"\")"=w180) -> ("States Out"=w179:string)  [unwired: 14 in]
      }
      frame Default {
        w190 = 42 items=["No error", "Argument error", "Memory is full", "Out of zone", "End of file", "File already open", "Generic file I/O error", "File not found", "File permission error", "Disk is full", "Duplicate path", "Too many files open", "System feature not enabled", "Resource file not found", "Cannot add resource", "Resource not found", "Image not found", "Image memory error", "Pen does not exist", "Config type invalid", "Config token not found", "Config parse error", "Config memory error", "Bad external code format", "Bad external code offset", "External code not present", "Null window", "Destroy window error", "Null menu", "Print aborted", "Bad print record", "Print driver error", "Windows error during printing", "Memory error during printing", "Print dialog error", "Generic print error", "Invalid device refnum", "Device not found", "Device parameter error", "Device unit error", "Cannot open device", "Device call aborted", "Generic error", "Cancelled by user", "Object ID too low", "Object ID too high", "Object not in heap", "Unknown heap", "Unknown object (invalid DefProc)", "Unknown object (DefProc not in table)", "Message out of range", "Invalid (null) method", "Unknown message", "Manager call not supported", "Bad address", "Network operation in progress", "Network operation timed out", "Connection is busy", "Network attribute not supported", "Network error", "Address in use", "System out of memory", "Connection aborted", "Connection refused", "Not connected", "Already connected", "Connection closed", "Initialization error (interapplication manager)", "Bad occurrence", "Wait on unbound occurrence handler", "Occurrence queue overflow", "Datalog type conflict", "Unused", "Unrecognized type (interapplication manager)", "Memory corrupt", "Failed to make temporary DLL", "Old CIN version", "Drag socket not found", "Failed to load drop-object", "Failed to register OLE object", "Failed to release OLE object", "Format specifier type mismatch", "Unknown format specifier", "Too few format specifiers", "Too many format specifiers", "Scan failed", "Newer CIN version", "Error converting to variant", "Runtime menu error", "Password tampered", "Variant attribute not found", "Incompatible variant data type", "Event data is not available", "Event Store is not present", "Occurrence is not found", "Event Queue is not created", "Event info is not available", "Refnum passed is NULL", "Error retrieving Class GUID", "Error retrieving CoClass GUID", "Error retrieving TypeLib GUID.", "Bad built application magic bytes.", "Specific driver is different from the specific driver associated with the Logical Name.", "There is no session opened to the class driver.", "Max Error", "MAX - Error with config objects", "MAX - Error loading configuration", "MAX - Group not supported"]
        # "Current State"
        # "Do not delete, rename, or modify this frame.\n(this is used to capture unhandled states and typos)"
        # "Handle mistyped state name (developer tool)"
        n89 = Format Into String(format string="Software Exception: Unhandled State \"%s\"." ("message"), error in=w186, w181) -> (resulting string=w189:string, error out=w188:errorcluster)  [unwired: 1 in]
        n90 = call <vilib>:"Error Cluster From Error Code.vi"("show call chain? (False)"=TRUE, "error in (no error)"=w188, "error message (\"\")"=w189, "error code (0)"=w190) -> ("error out"=w187:errorcluster)  [unwired: 5 in]
        n91 = call <vilib>:"Add State(s) to Queue__jki_lib_state_machine.vi"("State(s) in (\"\")"=w185) -> ("States Out"=w184:string)  [unwired: 14 in]
      }
      frame "Initialize Core Data" {
        # "Do not delete, rename, or modify this frame.\n(this is used to determine panel behavior on exit)"
        # "originally closed?"
        # "exe?"
        # "If panel starts closed or is an EXE, then close it when we exit"
        n92 = property class="VI"() -> ("Front Panel.Open"=w199:bool)  [unwired: 2 in, 2 out]
        n93 = property class="App"() -> ("App.Kind"=w198:T5)  [unwired: 2 in, 2 out]
        n94 = control-ref of="Current VI Reference"() -> (w192:refnum<vi>)
        n95 = Not(x=w199) -> (.not. x?=w196:bool)
        n96 = Equal?(x=w198, y=T5."Run Time System" ("Application:Kind")) -> (x = y?=w195:bool)
        n97 = Or(x=w196, y=w195) -> (x .or. y?=w193:bool)
        n98 = Bundle By Name(cluster=w194, "Core.Current VI Reference"=w192, "Core.Close Panel on Exit?"=w193) -> (w201:T7)
        n99 = call <vilib>:"Add State(s) to Queue__jki_lib_state_machine.vi"("State(s) in (\"\")"=w203) -> ("States Out"=w202:string)  [unwired: 14 in]
      }
      frame "Error Handler" {
        # "Unhandled Error -- Display it"
        # "Handle any errors here.\nYou can also output any states to clean-up after errors occur"
        # "Clear error"
        n100 = call <vilib>:"General Error Handler.vi"("error in (no error)"=w205) -> ()  [unwired: 10 in, 5 out]
        n101 = call <vilib>:"Add State(s) to Queue__jki_lib_state_machine.vi"("State(s) in Front (\"\")"="/* Post Error States", "State(s) in (\"\")"=w209) -> ("States Out"=w208:string)  [unwired: 13 in]
      }
      frame "Exit" {
        # "Do not put any code in this frame.\n(No errors that occur here will be handled.)"
        n102 = call <vilib>:"Add State(s) to Queue__jki_lib_state_machine.vi"("State(s) in (\"\")"=w214) -> ("States Out"=w213:string)  [unwired: 14 in]
      }
      frame "---------- Data ----------" {
        # "Do not put any code in this frame.\n(It is a separator no-op. You can make a copy of this frame to create a new Data frame)"
        n103 = call <vilib>:"Add State(s) to Queue__jki_lib_state_machine.vi"("State(s) in (\"\")"=w218) -> ("States Out"=w217:string)  [unwired: 14 in]
      }
      frame "Data: Initialize" {
        w219 = TRUE  # Open Gaia north shutter
        w220 = TRUE  # Open Gaia north shutter
        w221 = FALSE  # Gaia shutter enable
        w222 = TRUE  # IR beam on target
        w223 = TRUE  # auto purge
        w224 = FALSE  # purge
        w225 = 0  # jet status tck
        w226 = FALSE  # Phosphor enable
        w227 = FALSE  # Wedge enable
        w228 = FALSE  # Jet enable
        w229 = FALSE  # Fire Continues Allowed
        w231 = u32 0  # Jet probe stage tck
        w230 = u32 0  # Tik2
        w232 = FALSE  # Jet trigger
        w233 = 0.0  # ACavePressure
        w234 = 0.0  # BCavePressure
        w235 = T8 {"Current VI Reference"=refnum, "Close Panel on Exit?"=FALSE}  # Core
        # "do not delete - used by framework"
        # "Expand Bundle to add new data elements to shift register data."
        # "Add new data here."
        # "Data names and types of shift register data are defined by this bundle."
        # "Initialize the shift-register data, here.\n(data names are defined by what you wire into the bundle function)"
        n104 = Bundle("Core"=w235, "BCavePressure"=w234, "ACavePressure"=w233, "Jet trigger"=w232, "Jet probe stage tck"=w231, "Tik2"=w230, "Fire Continues Allowed"=w229, "Jet enable"=w228, "Wedge enable"=w227, "Phosphor enable"=w226, "jet status tck"=w225, "purge"=w224, "auto purge"=w223, "IR beam on target"=w222, "Gaia shutter enable"=w221, "Open Gaia north shutter"=w220, "Open Gaia north shutter"=w219) -> (w237:T7)  [unwired: 1 in]
        n105 = call <vilib>:"Add State(s) to Queue__jki_lib_state_machine.vi"("State(s) in (\"\")"=w239) -> ("States Out"=w238:string)  [unwired: 14 in]
      }
      frame "Data: Cleanup" {
        # "Cleanup any data and references, here.\n(this is called automatically, by the Macro: Exit)"
        n106 = Unbundle By Name(w240) -> ("Core.Current VI Reference"=w243:refnum<vi>)
        n107 = Close Reference(reference=w243, error in (no error)=w242) -> (error out=w241:errorcluster)
        n108 = call <vilib>:"Add State(s) to Queue__jki_lib_state_machine.vi"("State(s) in (\"\")"=w245) -> ("States Out"=w244:string)  [unwired: 14 in]
      }
      frame "---------- UI ----------" {
        # "Do not put any code in this frame.\n(It is a separator no-op. You can make a copy of this frame to create a new UI frame)"
        n109 = call <vilib>:"Add State(s) to Queue__jki_lib_state_machine.vi"("State(s) in (\"\")"=w249) -> ("States Out"=w248:string)  [unwired: 14 in]
      }
      frame "UI: Initialize" {
        # "Initialize the User Interface, here.\n(this is called automatically, by the Macro: Init)"
        n110 = call <vilib>:"Add State(s) to Queue__jki_lib_state_machine.vi"("State(s) in (\"\")"=w253) -> ("States Out"=w252:string)  [unwired: 14 in]
      }
      frame "UI: Cursor Set" {
        # "Argument"
        # "Set and Unset Cursor Busy.\n(Usage: \"UI: Cursor Set >> Busy|Idle\")"
        n111 = case shown="\"Idle\", Default" w254 {
          tunnel: w256 -> [w261 w263]
          tunnel: [w260 w262] -> w255
          frame "Idle", Default {
            n112 = call <vilib>:"Unset Busy.vi"("error in (no error)"=w261) -> ("error out"=w260:errorcluster)  [unwired: 10 in]
          }
          frame "Busy" {
            n113 = call <vilib>:"Set Busy.vi"("error in (no error)"=w263) -> ("error out"=w262:errorcluster)  [unwired: 9 in, 1 out]
          }
        }
        n114 = call <vilib>:"Add State(s) to Queue__jki_lib_state_machine.vi"("State(s) in (\"\")"=w259) -> ("States Out"=w258:string)  [unwired: 14 in]
      }
      frame "UI: Front Panel State" {
        # "Argument"
        # "Set Front Panel Open or Closed\n(Usage: \"UI: Front Panel State >> Open|Close\")"
        n115 = Unbundle By Name(w266) -> ("Core.Current VI Reference"=w265:refnum<vi>)
        n116 = case shown="\"Close\"" w264 {
          tunnel: w268 -> [w274 w287]
          tunnel: [w276 w288] -> w267
          tunnel: w265 -> [w275 w285]
          frame "Open", Default {
            n117 = property class="VI"(reference=w275, error in=w274) -> (reference out=w272:refnum<vi>, error out=w273:errorcluster, "Front Panel.Open"=w271:bool)
            n118 = case shown="False" w271 {
              tunnel: [w279 w282] -> w276
              tunnel: w273 -> [w278 w282]
              tunnel: w272 -> [w277 _]
              frame False {
                n119 = invoke class="VI" method="FP.Open"(reference=w277, error in=w278, "Activate"=TRUE, "State"=T6."Standard") -> (error out=w279:errorcluster)  [unwired: 1 in, 4 out]
              }
              frame True {
              }
            }
          }
          frame "Close" {
            n120 = property class="VI"(reference=w285, error in=w287) -> (reference out=w284:refnum<vi>, error out=w286:errorcluster, "Front Panel.Open"=w283:bool)
            n121 = case shown="True" w283 {
              tunnel: [w289 w292] -> w288
              tunnel: w286 -> [w289 w291]
              tunnel: w284 -> [_ w290]
              frame False {
              }
              frame True {
                n122 = invoke class="VI" method="FP.Close"(reference=w290, error in=w291) -> (error out=w292:errorcluster)  [unwired: 1 in, 2 out]
              }
            }
          }
        }
        n123 = call <vilib>:"Add State(s) to Queue__jki_lib_state_machine.vi"("State(s) in (\"\")"=w270) -> ("States Out"=w269:string)  [unwired: 14 in]
      }
      frame "---------- Macro ----------" {
        # "Do not put any code in this frame.\n(It is a separator no-op. You can make a copy of this frame to create a new Macro frame)"
        n124 = call <vilib>:"Add State(s) to Queue__jki_lib_state_machine.vi"("State(s) in (\"\")"=w296) -> ("States Out"=w295:string)  [unwired: 14 in]
      }
      frame "Macro: Initialize" {
        w297 = "Data: Initialize\nInitialize Core Data\nUI: Initialize\nUI: Front Panel State >> Open"  # Data: Initialize Initialize Core Data UI: Initialize UI: Front Panel State >> Open
        # "Initialization Macro\n(This is called once, when the VI starts)"
        n125 = call <vilib>:"Add State(s) to Queue__jki_lib_state_machine.vi"("State(s) in Front (\"\")"=w297, "State(s) in (\"\")"=w301) -> ("States Out"=w300:string)  [unwired: 13 in]
      }
      frame "Macro: Exit" {
        # "Exit Macro\n(This is called once, when the VI exits)"
        n126 = Unbundle By Name(w308) -> ("Core.Close Panel on Exit?"=w307:bool)
        n127 = Select(t="UI: Front Panel State >> Close", s=w307, f="") -> (s? t:f=w304:string)
        n128 = call <vilib>:"Add State(s) to Queue__jki_lib_state_machine.vi"("State(s) in (\"\")"=w304, "State(s) at Back (\"\")"="Data: Cleanup\nExit") -> ("States Out"=w302:string)  [unwired: 13 in]
        n129 = call <vilib>:"Add State(s) to Queue__jki_lib_state_machine.vi"("State(s) in Front (\"\")"=w302, "State(s) in (\"\")"=w311) -> ("States Out"=w310:string)  [unwired: 13 in]
      }
      frame "---------- New Category ----------" {
        # "Template Separator\n(You can make a copy of, or modify, this frame)"
        n130 = call <vilib>:"Add State(s) to Queue__jki_lib_state_machine.vi"("State(s) in (\"\")"=w315) -> ("States Out"=w314:string)  [unwired: 14 in]
      }
      frame "Action: Fire" {
        # "Your code here.\n(You can make a copy of, or modify, this frame)"
        n131 = property on="fire::10" class="Str"(error in=w317, "Val(Sgnl)"="fire>>force" ("Value (Signaling)")) -> (error out=w316:errorcluster)  [unwired: 1 in, 1 out]
        n132 = call <vilib>:"Add State(s) to Queue__jki_lib_state_machine.vi"("State(s) in (\"\")"=w321) -> ("States Out"=w320:string)  [unwired: 14 in]
      }
      frame "CheckJetTriggerAmp" {
        # "Your code here.\n(You can make a copy of, or modify, this frame)"
        n133 = Greater?(x="Amplitude.Ch AB::10", y=2.0) -> (0:w327:bool)
        n134 = property on="Position.Channel 3::1" class="Enum (strict)"() -> ("Value"=w323:T1)  [unwired: 2 in, 2 out]
        n135 = property on="Position.Channel 9::1" class="Enum (strict)"() -> ("Value"=w326:T1)  [unwired: 2 in, 2 out]
        n136 = case shown="True" w327 {
          tunnel: [FALSE TRUE] -> w324
          frame False {
          }
          frame True {
          }
        }
        n137 = local write "Jet trigger"(w324) -> ()
        n138 = case shown="\"Removed\", Default" w323 {
          tunnel: [TRUE FALSE] -> w322
          frame "Removed", Default {
          }
          frame "Inserted" {
          }
        }
        n139 = case shown="\"Removed\", Default" w326 {
          tunnel: [TRUE FALSE] -> w325
          frame "Removed", Default {
          }
          frame "Inserted" {
          }
        }
        n140 = local write "Open Gaia North Shutter"(w322) -> ()
        n141 = local write "Laser on target"(w325) -> ()
        n142 = Bundle By Name(cluster=w331, "Jet trigger"=w324, "IR beam on target"=w325, "Open Gaia north shutter"=w322) -> (w330:T7)
        n143 = call <vilib>:"Add State(s) to Queue__jki_lib_state_machine.vi"("State(s) in (\"\")"=w334) -> ("States Out"=w333:string)  [unwired: 14 in]
      }
      frame "CheckJetOpeningTime" {
        # "Your code here.\n(You can make a copy of, or modify, this frame)"
        n144 = Greater?(x="Delay.Ch B::10", y=1e-05) -> (0:w344:bool)
        n145 = case shown="True" w344 {
          tunnel: [w351 w352] -> w343
          tunnel: [w351 w352] -> w342
          frame False {
            w351 = FALSE
          }
          frame True {
            w352 = TRUE
          }
        }
        n146 = Bundle By Name(cluster=w347, "Jet enable"=w343) -> (w346:T7)
        n147 = local write "Jet enable"(w342) -> ()
        n148 = call <vilib>:"Add State(s) to Queue__jki_lib_state_machine.vi"("State(s) in (\"\")"=w350) -> ("States Out"=w349:string)  [unwired: 14 in]
      }
      frame "CheckPurgeValve" {
        # "Your code here.\n(You can make a copy of, or modify, this frame)"
        n149 = Equal?(x="SoftwareVars.Ch1::22", y=enum16{"off", "on"}."on") -> (x = y?=w356:bool)
        n150 = case shown="True" w356 {
          tunnel: [w366 w367] -> w353
          tunnel: [w366 w367] -> w357
          frame False {
            w366 = FALSE
          }
          frame True {
            w367 = TRUE
          }
        }
        n151 = Unbundle By Name(w361) -> ("Jet trigger"=w363:bool, "Jet enable"=w362:bool)
        n152 = local write "auto purge"(w357) -> ()
        n153 = case shown="True" w353 {
          tunnel: w363 -> [_ w384]
          tunnel: w362 -> [_ w383]
          tunnel: w361 -> [w373 w382]
          tunnel: [w372 w381] -> w360
          tunnel: w359 -> [w369 w378]
          tunnel: [w368 w377] -> w358
          frame False {
            n154 = property on="DO.Ch6::22" class="Enum (strict)"(error in=w369) -> (error out=w368:errorcluster, "Value"=w370:enum16{"off", "on"})  [unwired: 1 in, 1 out]
            n155 = case shown="\"on\"" w370 {
              tunnel: [w375 w376] -> w371
              tunnel: [w375 w376] -> w374
              frame "off", Default {
                w375 = FALSE
              }
              frame "on" {
                w376 = TRUE
              }
            }
            n156 = local write "purge"(w374) -> ()
            n157 = Bundle By Name(cluster=w373, "purge"=w371) -> (w372:T7)
          }
          frame True {
            n158 = And(x=w384, y=w383) -> (x .and. y?=w379:bool)
            n159 = case shown="False" w379 {
              tunnel: [w389 w399] -> w380
              tunnel: [w389 w399] -> w385
              tunnel: w378 -> [w387 w397]
              tunnel: [w390 w395] -> w377
              frame False {
                w389 = FALSE
                n160 = property on="DO.Ch6::22" class="Enum (strict)"(error in=w387) -> (error out=w386:errorcluster, "Value"=w388:enum16{"off", "on"})  [unwired: 1 in, 1 out]
                n161 = case shown="\"on\"" w388 {
                  tunnel: w386 -> [w391 w394]
                  tunnel: [w391 w393] -> w390
                  frame "off", Default {
                  }
                  frame "on" {
                    n162 = property on="DO.Ch6::22" class="Enum (strict)"(error in=w394, "Val(Sgnl)"=enum16{"off", "on"}."off" ("Value (Signaling)")) -> (error out=w393:errorcluster)  [unwired: 1 in, 1 out]
                  }
                }
              }
              frame True {
                w399 = TRUE
                n163 = property on="DO.Ch6::22" class="Enum (strict)"(error in=w397) -> (error out=w396:errorcluster, "Value"=w398:enum16{"off", "on"})  [unwired: 1 in, 1 out]
                n164 = case shown="\"off\", Default" w398 {
                  tunnel: w396 -> [w401 w403]
                  tunnel: [w400 w403] -> w395
                  frame "off", Default {
                    n165 = property on="DO.Ch6::22" class="Enum (strict)"(error in=w401, "Val(Sgnl)"=enum16{"off", "on"}."on" ("Value (Signaling)")) -> (error out=w400:errorcluster)  [unwired: 1 in, 1 out]
                  }
                  frame "on" {
                  }
                }
              }
            }
            n166 = Bundle By Name(cluster=w382, "purge"=w380) -> (w381:T7)
            n167 = local write "purge"(w385) -> ()
          }
        }
        n168 = call <vilib>:"Add State(s) to Queue__jki_lib_state_machine.vi"("State(s) in (\"\")"=w365) -> ("States Out"=w364:string)  [unwired: 14 in]
      }
      frame "UpdatePressure" {
        w412 = 1
        # "Your code here.\n(You can make a copy of, or modify, this frame)"
        n169 = for {
          N: w412 -> [_]
          tunnel: [w419] -> w415 mode=indexing
          tunnel: [w418] -> w404 mode=indexing
          n170 = local read "AI_mean.Channel 0::27"() -> (w419:dbl)
          n171 = Wait (ms)(milliseconds to wait=u32 2) -> ()  [unwired: 1 out]
          n172 = local read "AI_mean.Channel 1::27"() -> (w418:dbl)
        }
        n173 = Add Array Elements(numeric array=w415) -> (sum=w414:dbl)
        n174 = Divide(x=w414, y=w412) -> (x/y=w411:dbl)
        n175 = Add Array Elements(numeric array=w404) -> (sum=w413:dbl)
        n176 = call "pressure calibration.vi"("input variable"=w411) -> ("output variable"=w410:dbl)  [unwired: 10 in]
        n177 = Divide(x=w413, y=w412) -> (x/y=w409:dbl)
        n178 = call "pressure calibration.vi"("input variable"=w409) -> ("output variable"=w408:dbl)  [unwired: 10 in]
        n179 = Bundle By Name(cluster=w406, "BCavePressure"=w410, "ACavePressure"=w408) -> (w405:T7)
        n180 = call <vilib>:"Add State(s) to Queue__jki_lib_state_machine.vi"("State(s) in (\"\")"=w417) -> ("States Out"=w416:string)  [unwired: 14 in]
      }
    }
  }
